vi "BRig_dataTrial_Cue2_iTrial_1B.vi"() -> (2 "output_Cue2_iTrial_1B":i32)   [LabVIEW 2014]
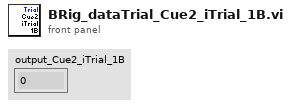
[diagram p1: front panel]
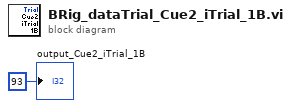
[diagram p0: block diagram]
diagram:
  "output_Cue2_iTrial_1B" <- 93 ("output_iBlock")
